vi "LoadProfilePowerTestK2Jarrett.vi"() -> ()   [LabVIEW 2020]
uses:
  <instrlib>/NH Research Regenerative Test Series/Public/Configure/Output Safety.ctl
  <vilib>/DAQmx/read.llb/DAQmx Read (Analog 1D DBL NChan 1Samp).vi
  <vilib>/Utility/file.llb/Read Delimited Spreadsheet (DBL).vi
  <instrlib>/NH Research Regenerative Test Series/Public/Data/Read (Ave Current).vi
  <instrlib>/NH Research Regenerative Test Series/Public/Data/Low Level/Fetch (Ave Voltage).vi
  <instrlib>/NH Research Regenerative Test Series/Public/Data/Low Level/Fetch (Ave True Power).vi
  <vilib>/DAQmx/miscellaneous.llb/DAQmx Fill In Error Info.vi
  <instrlib>/NH Research Regenerative Test Series/NH Research Regenerative Test Series.lvlib
panel:
  in  "Voltage Setpoint (0 V)":dbl format="%#.6g"
  out "first row 2":dbl[](array[numeric])
  out "first row":dbl[](array[numeric])
  in  "file path (dialog if empty) 2":path
  in  "file path (dialog if empty)":path
  out "Total Power":dbl
  out "Current Step":u32
  out "Time  Elapsed":dbl
  out "Time Step":dbl
  out "Load Output (A)":dbl
  out "Time Ref":dbl
  out "Control Power":dbl
  in  "Test Time (s)":dbl format="%#.6g"
  out "BatteryTempInternal":dbl
  out "BatteryWaterOut":dbl
  out "BatteryWaterIn":dbl
  out "Task error out":errorcluster
  out "String":string
  in  "Output Safety":T1
  out "Filename Out":path
  in  "DAQmx Task Name":refnum<k21>
  out "Ave Current (A)":dbl
  out "Ave Voltage (V)":dbl
  out "Ave True Power (W)":dbl
  out "Status Byte Register":T2
  in  "Logical Instrument Number":u32=1
  in  "Battery Detect Voltage (0V)":dbl format="%#.6g"
  in  "VISA resource name":refnum<visa-resource-name>
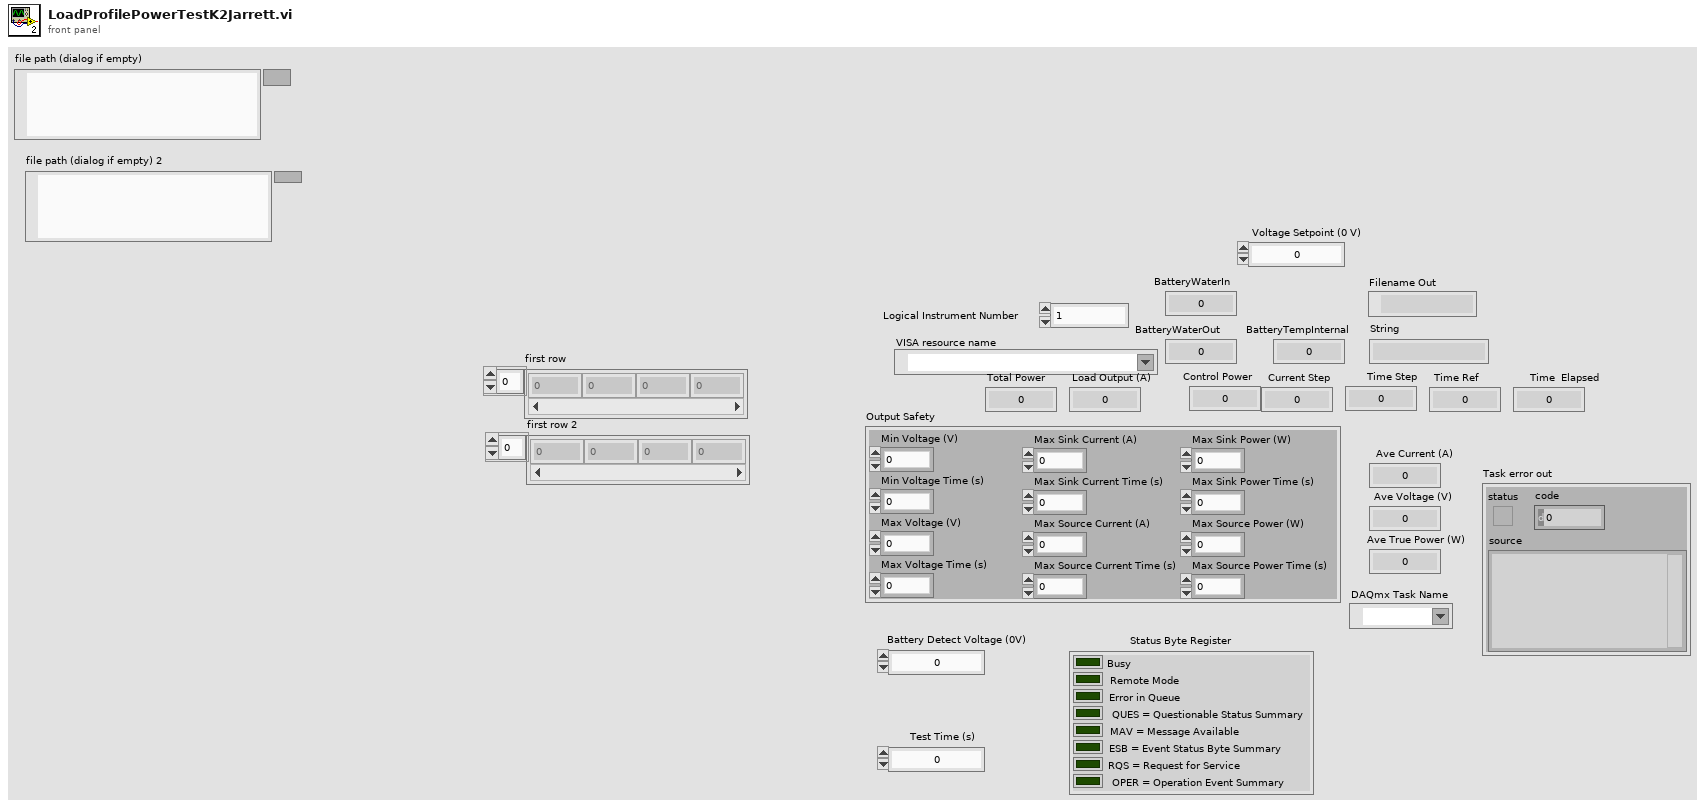
[diagram p1: front panel]
types:
  T1 = typedef "NH Research Regenerative Test Series.lvlib/Output Safety.ctl" = cluster{"Min Voltage (V)":dbl, "Min Voltage Time (s)":dbl, "Max Voltage (V)":dbl, "Max Voltage Time (s)":dbl, "Max Sink Current (A)":dbl, "Max Sink Current Time (s)":dbl, "Max Source Current (A)":dbl, "Max Source Current Time (s)":dbl, "Max Sink Power (W)":dbl, "Max Sink Power Time (s)":dbl, "Max Source Power (W)":dbl, "Max Source Power Time (s)":dbl}
  T2 = cluster{"Busy":bool, "Remote Mode":bool, "Error in Queue":bool, "QUES = Questionable Status Summary":bool, "MAV = Message Available":bool, "ESB = Event Status Byte Summary":bool, "RQS = Request for Service":bool, "OPER = Operation Event Summary":bool}
  T3 = cluster{"data[0]":dbl, "data[1]":dbl, "data[2]":dbl, "data[3]":dbl, "data[4]":dbl, "data[5]":dbl, "data[6]":dbl, "data[7]":dbl, "data[8]":dbl}
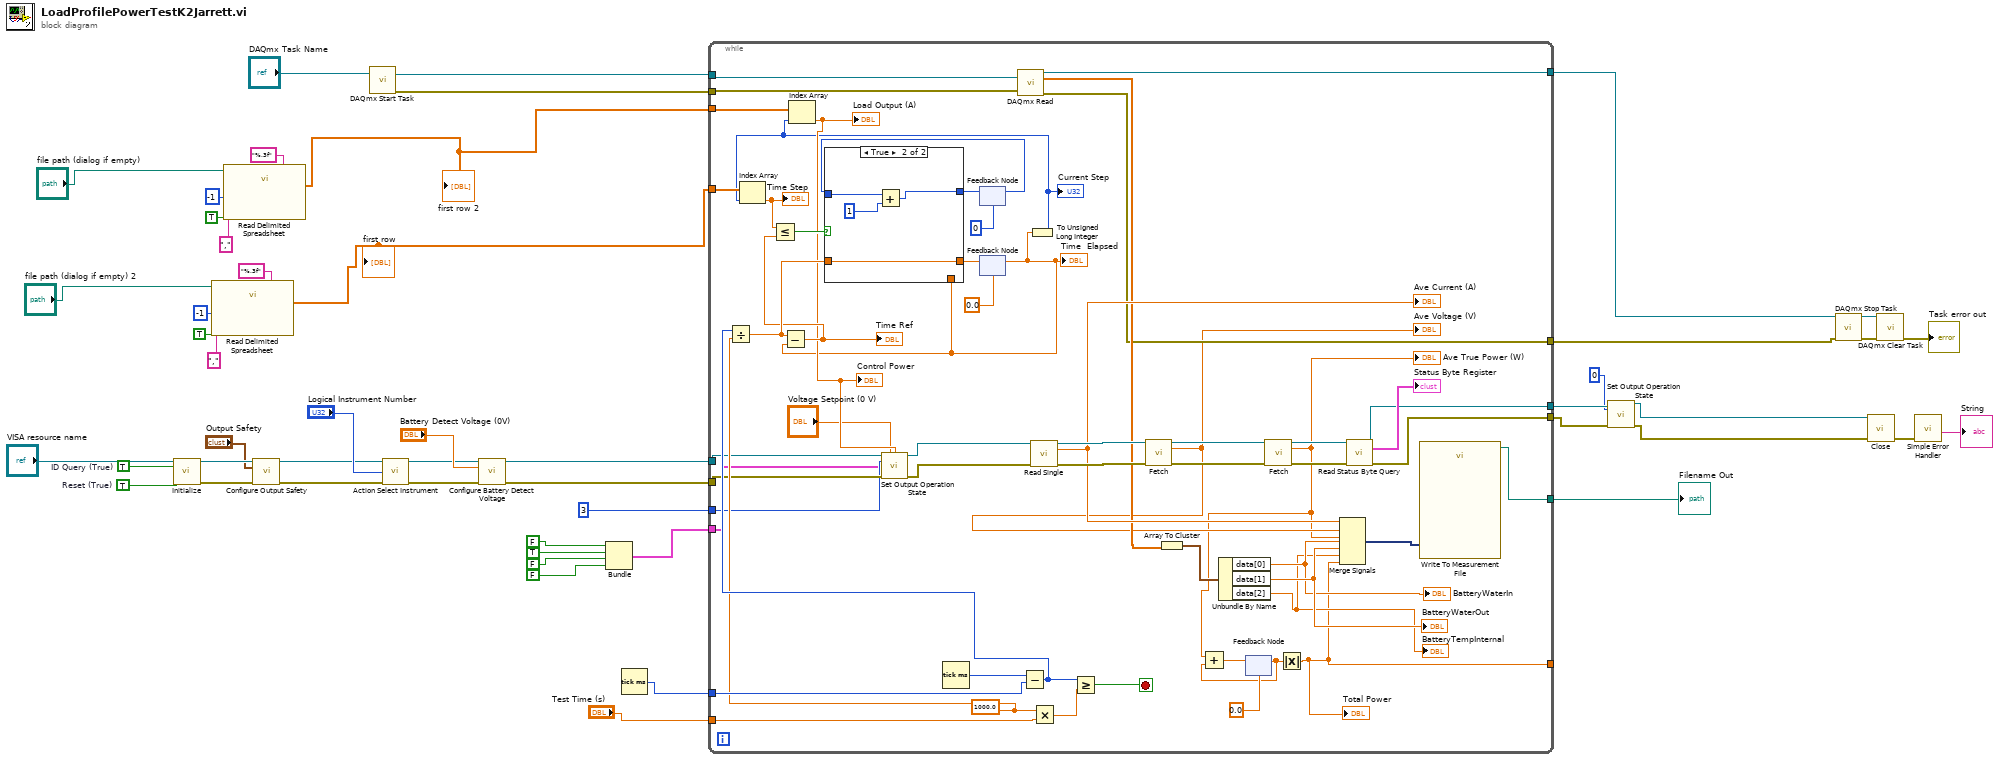
[diagram p0: block diagram]
diagram:
  w45 = TRUE  # ID Query (True)
  w44 = TRUE  # Reset (True)
  n1 = call <vilib>:"Initialize.vi"("VISA resource name"="VISA resource name", "ID Query (True)"=w45, "Reset (True)"=w44) -> ("VISA resource name out"=w43:refnum<visa-resource-name>, "error out"=w42:errorcluster)  [unwired: 11 in]
  n2 = call-poly <vilib>:"Read Delimited Spreadsheet.vi"("file path (dialog if empty)"="file path (dialog if empty) 2", "format (%.3f)"="%.3f", "number of rows (all:-1)"=-1, "transpose? (F)"=TRUE, "delimiter (\\t)"="," ("delimiter (\\t)")) -> ("first row"=w2:dbl[])  [unwired: 5 in, 5 out]
  "first row" <- w2
  n3 = call-poly <vilib>:"Read Delimited Spreadsheet.vi"("file path (dialog if empty)"="file path (dialog if empty)", "format (%.3f)"="%.3f", "number of rows (all:-1)"=-1, "transpose? (F)"=TRUE, "delimiter (\\t)"="," ("delimiter (\\t)")) -> ("first row"=w1:dbl[])  [unwired: 5 in, 5 out]
  "first row 2" <- w1
  n4 = call <vilib>:"Configure Output Safety.vi"("VISA resource name"=w43, "Output Safety"="Output Safety", "error in (no error)"=w42) -> ("VISA resource name out"=w39:refnum<visa-resource-name>, "error out"=w28:errorcluster)  [unwired: 11 in]
  n5 = call <vilib>:"DAQmx Start Task.vi"("task/channels in"="DAQmx Task Name") -> ("task out"=w37:refnum<k21>, "error out"=w29:errorcluster)  [unwired: 13 in]
  n6 = call <instrlib>:"Action Select Instrument.vi"("VISA resource name"=w39, "Logical Instrument Number"="Logical Instrument Number", "error in (no error)"=w28) -> ("VISA resource name out"=w49:refnum<visa-resource-name>, "error out"=w48:errorcluster)  [unwired: 11 in]
  n7 = call <vilib>:"Configure Battery Detect Voltage.vi"("VISA resource name"=w49, "Battery Detect Voltage (0V)"="Battery Detect Voltage (0V)", "error in (no error)"=w48) -> ("VISA resource name out"=w26:refnum<visa-resource-name>, "error out"=w25:errorcluster)  [unwired: 11 in]
  n8 = Bundle(FALSE, TRUE, FALSE, FALSE) -> (w20:cluster{bool, bool, bool, bool})  [unwired: 1 in]
  n9 = Tick Count (ms)() -> (millisecond timer value=w27:u32)
  n10 = while {
    tunnel: [w98] -> w17
    tunnel: [w97] -> w15
    tunnel: w37 -> [w95]
    tunnel: [w91] -> w31
    tunnel: [w90] -> w30
    tunnel: w29 -> [w89]
    tunnel: [w88] -> w46
    tunnel: w27 -> [w84]
    tunnel: "Test Time (s)" -> [w83]
    tunnel: w26 -> [w62]
    tunnel: w25 -> [w61]
    tunnel: w20 -> [w59]
    tunnel: 3 -> [w60]
    tunnel: w1 -> [w71]
    tunnel: w2 -> [w70]
    tunnel: [w55] -> _
    stop <- w82 stop-if-true
    w68 = 1000.0
    n11 = Tick Count (ms)() -> (millisecond timer value=w85:u32)
    n12 = feedback #1(0) -> (w72:i32)
    n13 = feedback #2(0.0) -> (w52:dbl)
    "Time  Elapsed" <- w52
    n14 = call-poly <vilib>:"DAQmx Read.vi"("task/channels in"=w95, "error in"=w89) -> ("task out"=w91:refnum<k21>, "data"=w94:dbl[], "error out"=w90:errorcluster)  [unwired: 11 in]
    n15 = Subtract(x=w85, y=w84) -> (x-y=w74:u32)
    n16 = Divide(x=w74, y=w68) -> (x/y=w81:dbl)
    n17 = Subtract(x=w81, y=w52) -> (x-y=w77:dbl)
    "Time Ref" <- w77
    n18 = To Unsigned Long Integer(number=w52) -> (unsigned 32bit integer=w51:u32)
    "Current Step" <- w51
    n19 = Index Array(array=w70, index=w51) -> (element=w69:dbl)
    "Time Step" <- w69
    n20 = Less Or Equal?(x=w69, y=w77) -> (x <= y?=w78:bool)
    n21 = Index Array(array=w71, index=w51) -> (element=w54:dbl)
    "Control Power" <- w54
    "Load Output (A)" <- w54
    n22 = case shown="True" w78 {
      tunnel: w81 -> [_ w111]
      tunnel: [w107 w111] -> w80
      tunnel: w52 -> [w107 _]
      tunnel: [w106 w109] -> w79
      tunnel: w72 -> [w106 w108]
      frame False {
      }
      frame True {
        n23 = Add(x=w108, y=1) -> (x+y=w109:i32)
      }
    }
    n24 = call <vilib>:"Set Output Operation State.vi"("VISA resource name"=w62, "Voltage Setpoint (0 V)"="Voltage Setpoint (0 V)", "Current Setpoint (0 A)"=w54, "Mode (0: Off)"=w60, "Enable"=w59, "error in (no error)"=w61) -> ("VISA resource name out"=w63:refnum<visa-resource-name>, "error out"=w58:errorcluster)  [unwired: 8 in]
    n25 = feedback-in #1(w79) -> ()
    n26 = feedback-in #2(w80) -> ()
    n27 = call-poly <instrlib>:"Read Single.vi"("VISA resource name"=w63, "error in (no error)"=w58) -> ("VISA resource name out"=w104:refnum<visa-resource-name>, "Ave Current (A)"=w96:dbl, "error out"=w105:errorcluster)  [unwired: 11 in]
    "Ave Current (A)" <- w96
    n28 = Multiply(x=w68, y=w83) -> (x*y=w73:dbl)
    n29 = Greater Or Equal?(x=w74, y=w73) -> (x >= y?=w82:bool)
    n30 = call-poly <instrlib>:"Fetch.vi"("VISA resource name"=w104, "error in (no error)"=w105) -> ("VISA resource name out"=w103:refnum<visa-resource-name>, "Ave Voltage (V)"=w87:dbl, "error out"=w102:errorcluster)  [unwired: 11 in]
    "Ave Voltage (V)" <- w87
    n31 = Array To Cluster(array=w94) -> (cluster=w93:T3)
    n32 = Unbundle By Name(w93) -> ("data[0]"=w57:dbl, "data[1]"=w86:dbl, "data[2]"=w56:dbl)
    "BatteryWaterIn" <- w57
    "BatteryWaterOut" <- w86
    "BatteryTempInternal" <- w56
    n33 = feedback #3(0.0) -> (w64:dbl)
    n34 = call-poly <instrlib>:"Fetch.vi"("VISA resource name"=w103, "error in (no error)"=w102) -> ("VISA resource name out"=w101:refnum<visa-resource-name>, "Ave True Power (W)"=w65:dbl, "error out"=w100:errorcluster)  [unwired: 11 in]
    "Ave True Power (W)" <- w65
    n35 = Add(x=w65, y=w64) -> (x+y=w66:dbl)
    n36 = feedback-in #3(w66) -> ()
    n37 = Absolute Value(x=w64) -> (abs(x)=w55:dbl)
    "Total Power" <- w55
    n38 = Merge Signals "Merge Signals"(w96, w87, w65, w57, w86, w56, w55) -> (w92:dynamicdata)
    n39 = call <instrlib>:"Read Status Byte Query.vi"("VISA resource name"=w101, "error in (no error)"=w100) -> ("VISA resource name out"=w98:refnum<visa-resource-name>, "Status Byte Register"=→"Status Byte Register":T2, "error out"=w97:errorcluster)  [unwired: 11 in]
    n40 = call "Write To Measurement File"("Signals"=w92) -> ("Filename Out"=w88:path)  [unwired: 16 in, 2 out]
  }
  "Filename Out" <- w46
  n41 = call <vilib>:"Set Output Operation State.vi"("VISA resource name"=w17, "Mode (0: Off)"=0, "error in (no error)"=w15) -> ("VISA resource name out"=w14:refnum<visa-resource-name>, "error out"=w13:errorcluster)  [unwired: 11 in]
  n42 = call <vilib>:"DAQmx Stop Task.vi"("task/channels in"=w31, "error in"=w30) -> ("task out"=w35:refnum<k21>, "error out"=w34:errorcluster)  [unwired: 12 in]
  n43 = call <instrlib>:"Close.vi"("VISA resource name"=w14, "error in (no error)"=w13) -> ("error out"=w32:errorcluster)  [unwired: 13 in]
  n44 = call <vilib>:"DAQmx Clear Task.vi"("task in"=w35, "error in"=w34) -> ("error out"=→"Task error out":errorcluster)  [unwired: 13 in]
  n45 = call <vilib>:"Simple Error Handler.vi"("error in (no error)"=w32) -> ("source out"=→"String":string)  [unwired: 4 in, 4 out]
